vi "wheels.vi"(0 "Speed 4":dbl(slide) scale=0.0..10.0, 1 "Speed 3":dbl(slide) scale=0.0..10.0, 2 "Speed 2":dbl(slide) scale=0.0..10.0, 3 "Speed 1":dbl(slide) scale=0.0..10.0, 8 "Steer 4":dbl(knob) scale=-180.0..180.0, 9 "Steer 3":dbl(knob) scale=-180.0..180.0, 10 "Steer 2":dbl(knob) scale=-180.0..180.0, 11 "Steer 1":dbl(knob) scale=-180.0..180.0) -> ()   [LabVIEW 2023]
uses:
  <vilib>/Rock Robotics/WPI/ThirdParty/Phoenix-LabVIEW/CANCoder/Get/CTRE_Phoenix_CANcoder_GetSensorData.vi
panel:
  out "Absolute Position 4":dbl
  out "Absolute Position 3":dbl
  out "Absolute Position 2":dbl
  out "Absolute Position 1":dbl
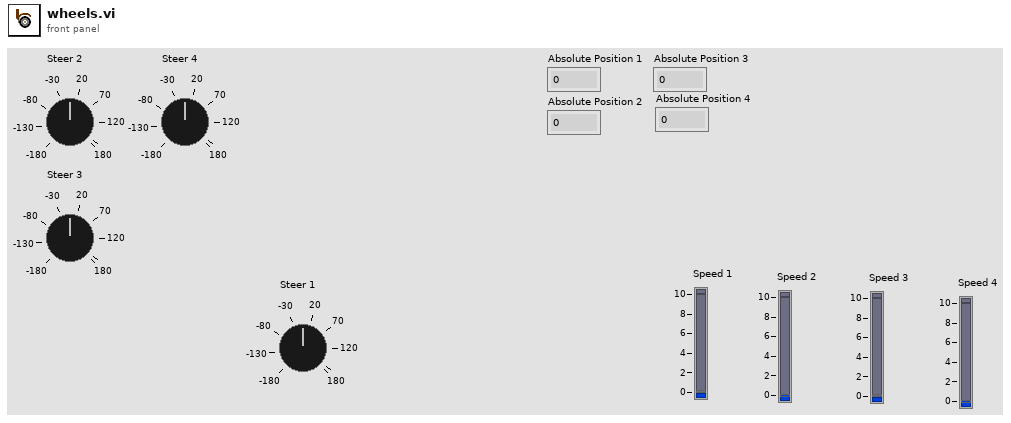
[diagram p1: front panel]
types:
  T1 = typedef "CTRE_Phoenix_CANcoder_DeviceRef.ctl" = cluster{"DeviceStatus":errorcluster, "Device Number":u8, "Handle":u64, "UsageFrame":u32, "Library Path":path}
  T2 = typedef "WPI_MotorControlDeviceRef.ctl" = cluster{"DeviceStatus":errorcluster, "Type":T3, "PWM":cluster{"PWM Channel":T4, "DeadBand":T5}, "CAN":cluster{"Device Number":u8, "SetOutput VI Ref":variant, "GetOutput VI Ref":variant, "Enable VI Ref":variant, "Disable VI Ref":variant, "Data":variant}, "Invert":bool, "DIO PWM":cluster{"PWM \"Enable\" Channel":T4, "DIOChannel":T6, "PWM Rate":dbl}}
  T3 = typedef "WPI_MotorControlType.ctl" = enum16{"PWM", "CAN", "DIO PWM"}
  T4 = typedef "FPGA_DIOPWMChannel.ctl" = enum8{"PWM 0", "PWM 1", "PWM 2", "PWM 3", "PWM 4", "PWM 5", "PWM 6", "PWM 7", "PWM 8", "PWM 9", "PWM MXP 0", "PWM MXP 1", "PWM MXP 2", "PWM MXP 3", "PWM MXP 4", "PWM MXP 5", "PWM MXP 6", "PWM MXP 7", "PWM MXP 8", "PWM MXP 9", "Invalid"}
  T5 = typedef "WPI_PWMDeadband.ctl" = cluster{"Name":string, "maxPositivePwm":i32, "minPositivePwm":i32, "centerPwm":i32, "maxNegativePwm":i32, "minNegativePwm":i32, "angularRange":u16}
  T6 = typedef "FPGA_DIOChannel.ctl" = enum8{"DIO 0", "DIO 1", "DIO 2", "DIO 3", "DIO 4", "DIO 5", "DIO 6", "DIO 7", "DIO 8", "DIO 9", "DIO MXP 0", "DIO MXP 1", "DIO MXP 2", "DIO MXP 3", "DIO MXP 4", "DIO MXP 5", "DIO MXP 6", "DIO MXP 7", "DIO MXP 8", "DIO MXP 9", "DIO MXP 10", "DIO MXP 11", "DIO MXP 12", "DIO MXP 13", "DIO MXP 14", "DIO MXP 15", "SPI Port CS1", "SPI Port CS2", "SPI Port CS3", "SPI Port MISO", "SPI Port MOSI", "Invalid"}
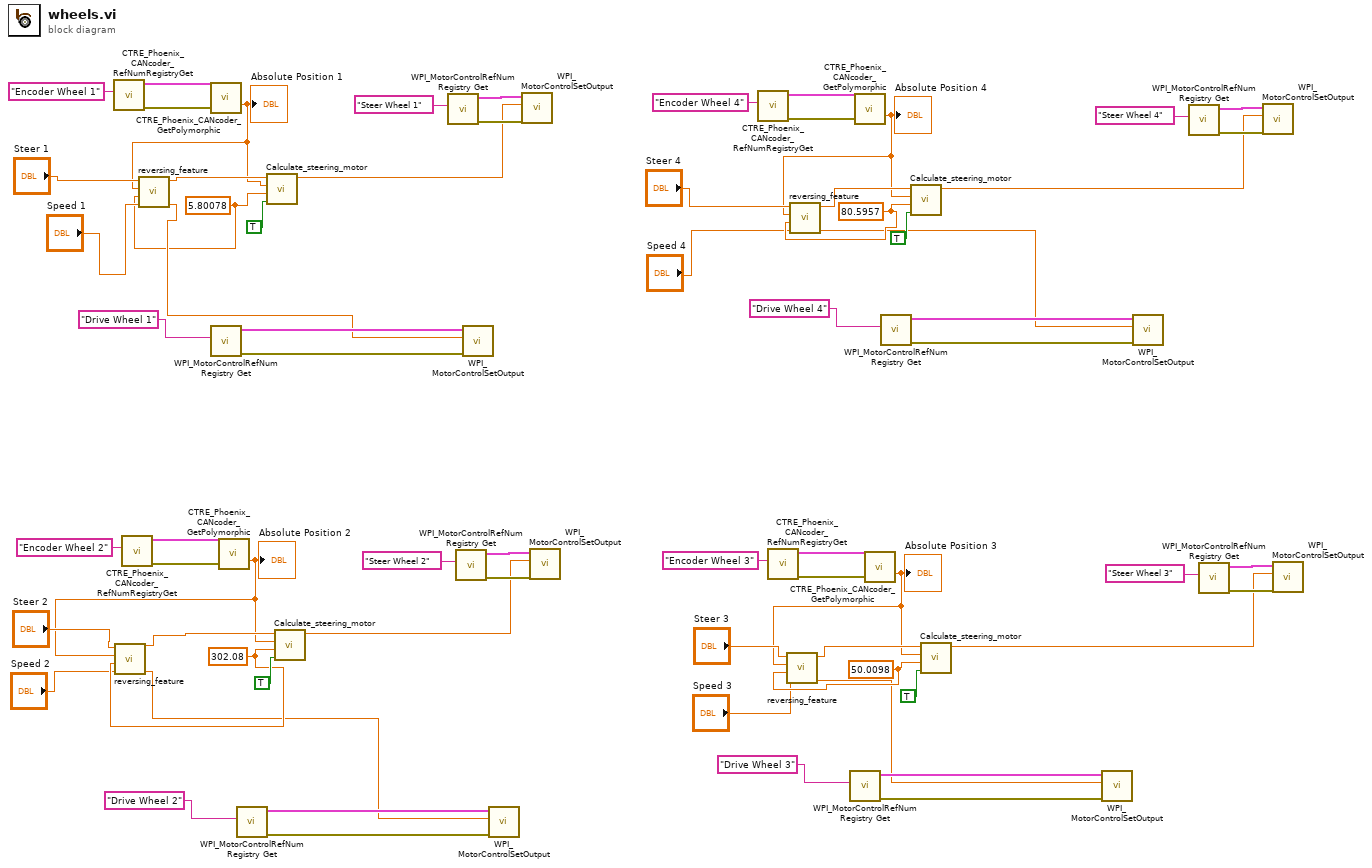
[diagram p0: block diagram]
diagram:
  w10 = 80.5957 ("Offset Angle")
  w7 = 50.0098 ("Offset Angle")
  w8 = 302.08 ("Offset Angle")
  w9 = 5.80078 ("Offset Angle")
  n1 = call <vilib>:"CTRE_Phoenix_CANcoder_RefNumRegistryGet.vi"("refnum name"="Encoder Wheel 1") -> ("error out"=w66:errorcluster, "CTRE_CANcoder_DeviceRef"=w67:T1)  [unwired: 9 in]
  n2 = call <vilib>:"CTRE_Phoenix_CANcoder_RefNumRegistryGet.vi"("refnum name"="Encoder Wheel 2") -> ("error out"=w58:errorcluster, "CTRE_CANcoder_DeviceRef"=w59:T1)  [unwired: 9 in]
  n3 = call-poly <vilib>:"CTRE_Phoenix_CANcoder_GetPolymorphic.vi"("CTRE_CANcoder_DeviceRef"=w67, "error in"=w66) -> ("Absolute Position"=w11:dbl)  [unwired: 9 in, 4 out]
  "Absolute Position 1" <- w11
  n4 = call "reversing_feature.vi"("speed in"="Speed 1", "offset angle"=w9, "meas angle in"=w11, "set angle in"="Steer 1") -> ("speed out"=w13:dbl, "set angle out"=w12:dbl)  [unwired: 6 in]
  n5 = call <vilib>:"WPI_MotorControlRefNum Registry Get.vi"("refnum name"="Drive Wheel 1") -> ("error out"=w34:errorcluster, "MotorControlDevRef"=w36:T2)  [unwired: 9 in]
  n6 = call-poly <vilib>:"CTRE_Phoenix_CANcoder_GetPolymorphic.vi"("CTRE_CANcoder_DeviceRef"=w59, "error in"=w58) -> ("Absolute Position"=w22:dbl)  [unwired: 9 in, 4 out]
  "Absolute Position 2" <- w22
  n7 = call "reversing_feature.vi"("speed in"="Speed 2", "offset angle"=w8, "meas angle in"=w22, "set angle in"="Steer 2") -> ("speed out"=w1:dbl, "set angle out"=w24:dbl)  [unwired: 6 in]
  n8 = call <vilib>:"WPI_MotorControlRefNum Registry Get.vi"("refnum name"="Drive Wheel 2") -> ("error out"=w32:errorcluster, "MotorControlDevRef"=w33:T2)  [unwired: 9 in]
  n9 = call "Calculate_steering_motor.vi"("Invert?"=TRUE, "Offset Angle"=w9, "Absolute Position"=w11, "Angle"=w12) -> ("Steering Motor Output"=w62:dbl)  [unwired: 6 in, 1 out]
  n10 = call "Calculate_steering_motor.vi"("Invert?"=TRUE, "Offset Angle"=w8, "Absolute Position"=w22, "Angle"=w24) -> ("Steering Motor Output"=w54:dbl)  [unwired: 6 in, 1 out]
  n11 = call <vilib>:"WPI_MotorControlRefNum Registry Get.vi"("refnum name"="Steer Wheel 1") -> ("error out"=w65:errorcluster, "MotorControlDevRef"=w64:T2)  [unwired: 9 in]
  n12 = call <vilib>:"WPI_MotorControlRefNum Registry Get.vi"("refnum name"="Steer Wheel 2") -> ("error out"=w57:errorcluster, "MotorControlDevRef"=w56:T2)  [unwired: 9 in]
  n13 = call <vilib>:"WPI_MotorControlSetOutput.vi"("error in (no error)"=w34, "Output"=w13, "MotorControlDevRef"=w36) -> ()  [unwired: 6 in, 3 out]
  n14 = call <vilib>:"WPI_MotorControlSetOutput.vi"("error in (no error)"=w32, "Output"=w1, "MotorControlDevRef"=w33) -> ()  [unwired: 6 in, 3 out]
  n15 = call <vilib>:"WPI_MotorControlSetOutput.vi"("error in (no error)"=w65, "Output"=w62, "MotorControlDevRef"=w64) -> ()  [unwired: 6 in, 3 out]
  n16 = call <vilib>:"WPI_MotorControlSetOutput.vi"("error in (no error)"=w57, "Output"=w54, "MotorControlDevRef"=w56) -> ()  [unwired: 6 in, 3 out]
  n17 = call <vilib>:"CTRE_Phoenix_CANcoder_RefNumRegistryGet.vi"("refnum name"="Encoder Wheel 4") -> ("error out"=w42:errorcluster, "CTRE_CANcoder_DeviceRef"=w43:T1)  [unwired: 9 in]
  n18 = call <vilib>:"CTRE_Phoenix_CANcoder_RefNumRegistryGet.vi"("refnum name"="Encoder Wheel 3") -> ("error out"=w50:errorcluster, "CTRE_CANcoder_DeviceRef"=w51:T1)  [unwired: 9 in]
  n19 = call <vilib>:"WPI_MotorControlRefNum Registry Get.vi"("refnum name"="Drive Wheel 3") -> ("error out"=w29:errorcluster, "MotorControlDevRef"=w30:T2)  [unwired: 9 in]
  n20 = call-poly <vilib>:"CTRE_Phoenix_CANcoder_GetPolymorphic.vi"("CTRE_CANcoder_DeviceRef"=w43, "error in"=w42) -> ("Absolute Position"=w16:dbl)  [unwired: 9 in, 4 out]
  "Absolute Position 4" <- w16
  n21 = call "reversing_feature.vi"("speed in"="Speed 4", "offset angle"=w10, "meas angle in"=w16, "set angle in"="Steer 4") -> ("speed out"=w5:dbl, "set angle out"=w17:dbl)  [unwired: 6 in]
  n22 = call-poly <vilib>:"CTRE_Phoenix_CANcoder_GetPolymorphic.vi"("CTRE_CANcoder_DeviceRef"=w51, "error in"=w50) -> ("Absolute Position"=w19:dbl)  [unwired: 9 in, 4 out]
  "Absolute Position 3" <- w19
  n23 = call "reversing_feature.vi"("speed in"="Speed 3", "offset angle"=w7, "meas angle in"=w19, "set angle in"="Steer 3") -> ("speed out"=w3:dbl, "set angle out"=w20:dbl)  [unwired: 6 in]
  n24 = call <vilib>:"WPI_MotorControlRefNum Registry Get.vi"("refnum name"="Drive Wheel 4") -> ("error out"=w26:errorcluster, "MotorControlDevRef"=w27:T2)  [unwired: 9 in]
  n25 = call "Calculate_steering_motor.vi"("Invert?"=TRUE, "Offset Angle"=w10, "Absolute Position"=w16, "Angle"=w17) -> ("Steering Motor Output"=w38:dbl)  [unwired: 6 in, 1 out]
  n26 = call "Calculate_steering_motor.vi"("Invert?"=TRUE, "Offset Angle"=w7, "Absolute Position"=w19, "Angle"=w20) -> ("Steering Motor Output"=w46:dbl)  [unwired: 6 in, 1 out]
  n27 = call <vilib>:"WPI_MotorControlSetOutput.vi"("error in (no error)"=w29, "Output"=w3, "MotorControlDevRef"=w30) -> ()  [unwired: 6 in, 3 out]
  n28 = call <vilib>:"WPI_MotorControlSetOutput.vi"("error in (no error)"=w26, "Output"=w5, "MotorControlDevRef"=w27) -> ()  [unwired: 6 in, 3 out]
  n29 = call <vilib>:"WPI_MotorControlRefNum Registry Get.vi"("refnum name"="Steer Wheel 4") -> ("error out"=w41:errorcluster, "MotorControlDevRef"=w40:T2)  [unwired: 9 in]
  n30 = call <vilib>:"WPI_MotorControlRefNum Registry Get.vi"("refnum name"="Steer Wheel 3") -> ("error out"=w49:errorcluster, "MotorControlDevRef"=w48:T2)  [unwired: 9 in]
  n31 = call <vilib>:"WPI_MotorControlSetOutput.vi"("error in (no error)"=w41, "Output"=w38, "MotorControlDevRef"=w40) -> ()  [unwired: 6 in, 3 out]
  n32 = call <vilib>:"WPI_MotorControlSetOutput.vi"("error in (no error)"=w49, "Output"=w46, "MotorControlDevRef"=w48) -> ()  [unwired: 6 in, 3 out]
